vi "Servo_serial_PositionCalibration.vi"() -> ()   [LabVIEW 2017]
uses:
  <vilib>/Instr/_visa.llb/VISA Configure Serial Port (Instr).vi
panel:
  out "Servo Digital Signal":cluster{i32, dbl, dbl[]}(graph)
  out "Position Input":cluster{i32, dbl, dbl[]}(graph)
  out "Digitial Signal":dbl
  in  "Sample Rate":dbl
  in  "Buad Rate":i32(ring) items=["2400"=2400, "4800"=4800, "9600"=9600, "14400"=14400, "19200"=19200, "28800"=28800, "38400"=38400, "57600"=57600, "115200"=115200]
  out "Bytes at port":cluster{i32, dbl, dbl[]}(graph)
  out "Read buffer":string
  in  "Stop":bool
  out "Sent to Arduino":string
  in  "COM Port":refnum<visa-resource-name>
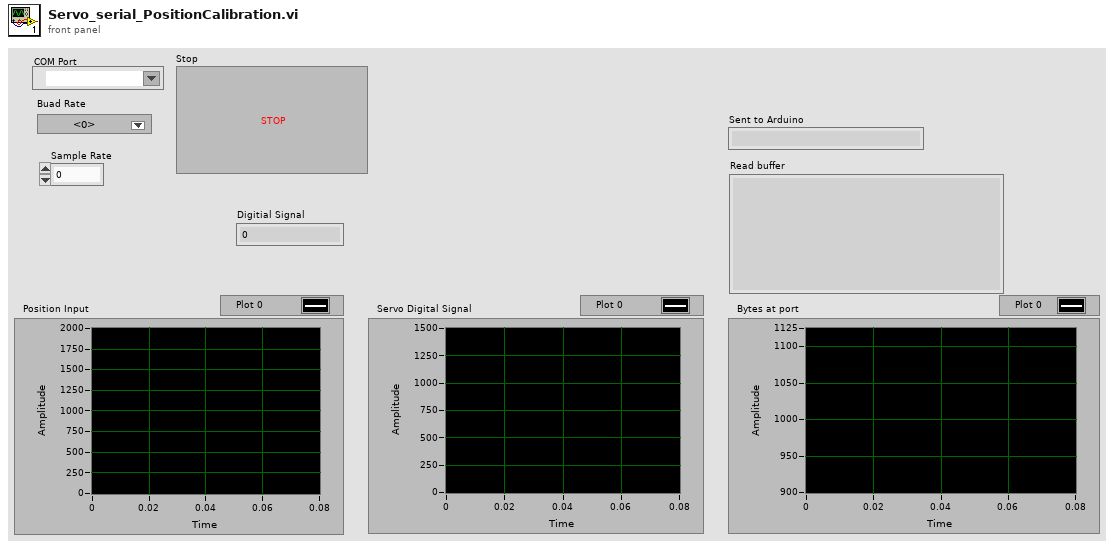
[diagram p1: front panel]
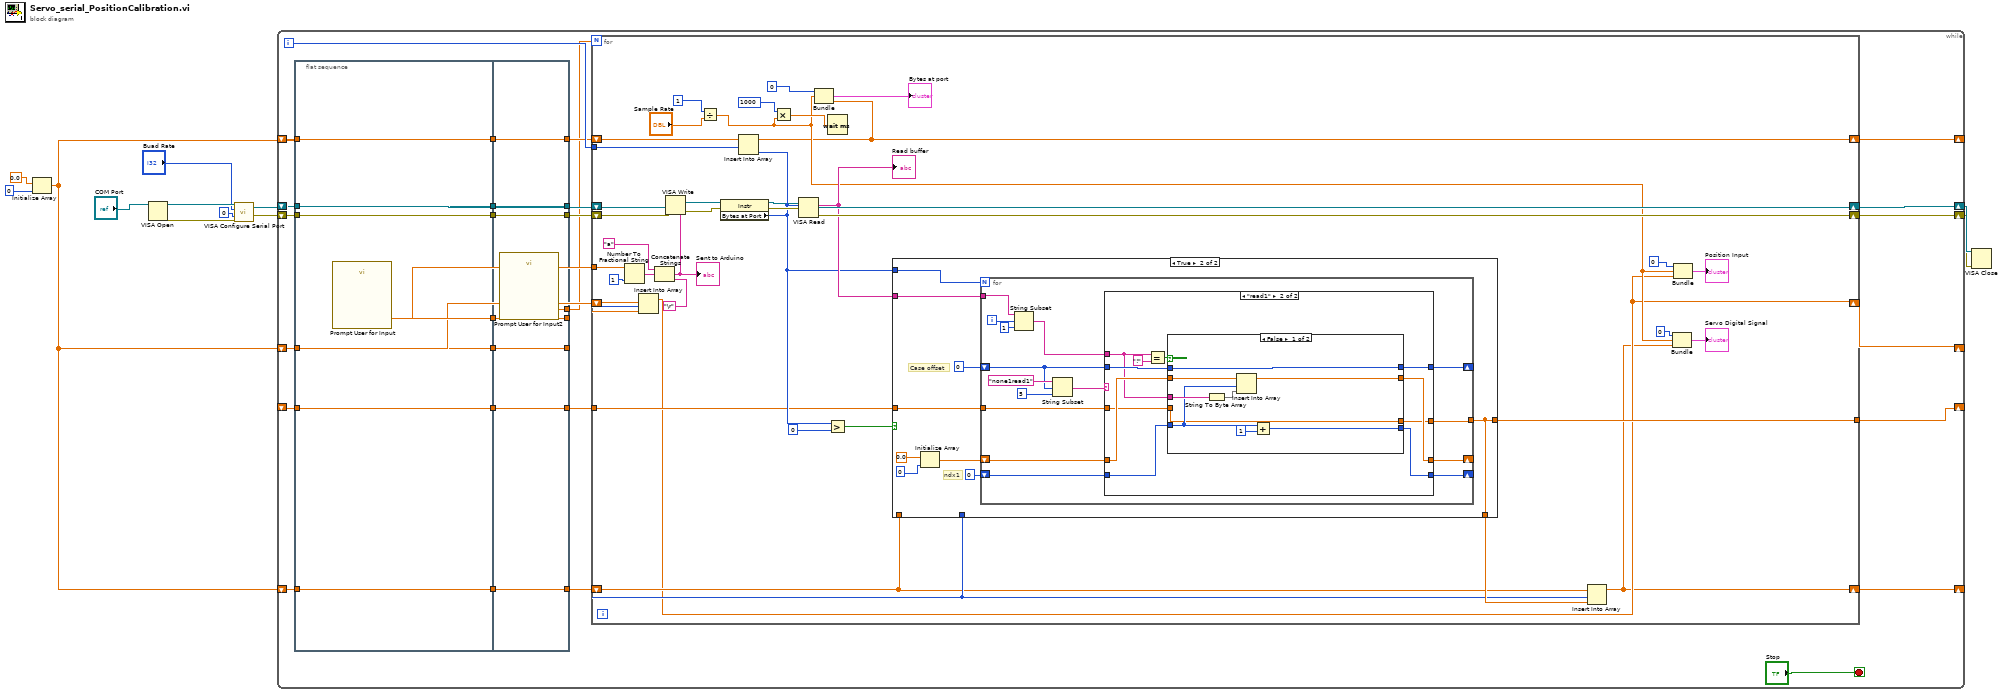
[diagram p0: block diagram]
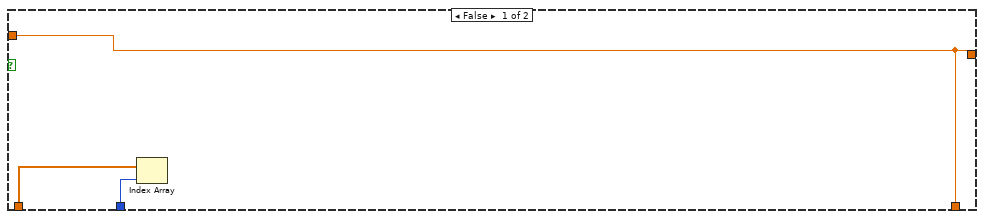
[diagram p2: hidden frame]
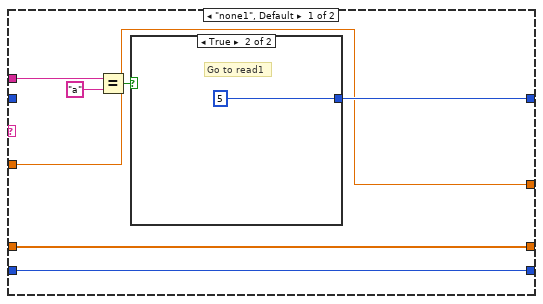
[diagram p3: hidden frame]
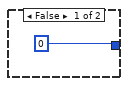
[diagram p4: hidden frame]
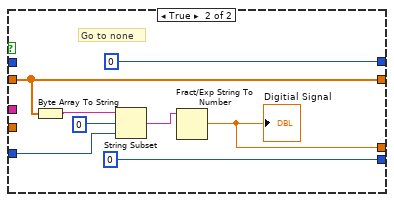
[diagram p5: hidden frame]
diagram:
  n1 = Initialize Array(0.0 ("element"), 0 ("dimension size")) -> (w7:dbl[])
  n2 = VISA Open(VISA resource name="COM Port") -> (VISA resource name=w6:refnum<visa-resource-name>, error out=w4:errorcluster)  [unwired: 4 in]
  n3 = call-poly "VISA Configure Serial Port"("VISA resource name"=w6, "baud rate (9600)"="Buad Rate", "parity (0:none)"=0, "error in (no error)"=w4) -> ("VISA resource name out"=w2:refnum<visa-resource-name>, "error out"=w3:errorcluster)  [unwired: 10 in]
  n4 = while {
    shift-right: [w36] -> w11
    shift-left: w2 -> [w30]
    shift-right: [w37] -> w10
    shift-left: w3 -> [w19]
    shift-right: [w18] -> _
    shift-left: w7 -> [w31]
    shift-right: [w17] -> _
    shift-left: w7 -> [w29]
    shift-right: [w16] -> _
    shift-left: w7 -> [w27]
    shift-right: [w32] -> _
    shift-left: _ -> [w28]
    i -> [w34]
    stop <- "Stop" stop-if-true
    n5 = flat-sequence {
      tunnel: w31 -> [w147]
      tunnel: w30 -> [w146]
      tunnel: w29 -> [w145]
      tunnel: w28 -> [w144]
      tunnel: w27 -> [w143]
      tunnel: [w142] -> w26
      tunnel: [w147] -> w25
      tunnel: [w146] -> w24
      tunnel: [w145] -> w23
      tunnel: [w144] -> w22
      tunnel: [w143] -> w21
      tunnel: [w141] -> w20
      tunnel: w19 -> [w141]
      tunnel: [w150] -> w13
      tunnel: [w151] -> w14
      tunnel: [w152] -> _
      tunnel: [w153] -> _
      tunnel: [w154] -> _
      tunnel: [w155] -> w33
      tunnel: w26 -> [w155]
      tunnel: w25 -> [w154]
      tunnel: w24 -> [w153]
      tunnel: w23 -> [w152]
      tunnel: w22 -> [w151]
      tunnel: w21 -> [w150]
      tunnel: [w149] -> _
      tunnel: w20 -> [w149]
      tunnel: [w148] -> w15
      frame #0 {
        n6 = call "Prompt User for Input"() -> ("Pulse Width"=w142:dbl)  [unwired: 17 in, 2 out]
      }
      frame #1 {
        n7 = call "Prompt User for Input2"() -> ("Number Of Trials"=w148:dbl)  [unwired: 17 in, 2 out]
      }
    }
    n8 = for {
      N: w15 -> [_]
      tunnel: w34 -> [w57]
      tunnel: w33 -> [w53]
      tunnel: [w52] -> w32
      tunnel: w14 -> [w43]
      shift-right: [w75] -> w36
      shift-left: w30 -> [w45]
      shift-right: [w76] -> w37
      shift-left: w19 -> [w41]
      shift-right: [w38] -> w16
      shift-left: w13 -> [w42]
      shift-right: [w39] -> w17
      shift-left: w29 -> [w44]
      shift-right: [w40] -> w18
      shift-left: w31 -> [w46]
      n9 = Number To Fractional String(number=w53, precision (6)=1) -> (F-format string=w73:string)  [unwired: 2 in]
      n10 = Insert Into Array(array=w44, index=w57, new element=w53) -> (w39:dbl[])
      n11 = Concatenate Strings("a", w73, "\r") -> (w74:string)
      "Sent to Arduino" <- w74
      n12 = VISA Write(VISA resource name=w45, write buffer=w74, error in (no error)=w41) -> (VISA resource name out=w68:refnum<visa-resource-name>, error out=w71:errorcluster)  [unwired: 1 out]
      n13 = Divide(x=1, y="Sample Rate") -> (x/y=w48:dbl)
      n14 = property class="Instr"(reference=w68, error in=w71) -> (reference out=w69:refnum<visa-resource-name>, error out=w70:errorcluster, "Bytes at Port"=w63:u32)
      n15 = Insert Into Array(array=w46, index=w57, new element=w63) -> (w40:dbl[])
      n16 = Multiply(x=1000, y=w48) -> (x*y=w49:dbl)
      n17 = VISA Read(VISA resource name=w69, byte count=w63, error in (no error)=w70) -> (VISA resource name out=w75:refnum<visa-resource-name>, read buffer=w65:string, error out=w76:errorcluster)  [unwired: 1 out]
      "Read buffer" <- w65
      n18 = Bundle(0, w48, w40) -> (→"Bytes at port":cluster{i32, dbl, dbl[]})  [unwired: 1 in]
      n19 = Wait (ms)(milliseconds to wait=w49) -> ()  [unwired: 1 out]
      n20 = Greater?(x=w63, y=0) -> (0:w62:bool)
      n21 = case shown="True" w62 {
        tunnel: w63 -> [_ w82]
        tunnel: w65 -> [_ w88]
        tunnel: [w77 w80] -> w58
        tunnel: w57 -> [w78 _]
        tunnel: w42 -> [w79 _]
        tunnel: w43 -> [w77 w81]
        tunnel: [w77 w80] -> w52
        frame False {
          n22 = Index Array(array=w79, index=w78) -> ()  [unwired: 1 out]
        }
        frame True {
          # "ndx1"
          # "Case offset"
          n23 = Initialize Array(0.0 ("element"), 0 ("dimension size")) -> (w83:dbl[])
          n24 = for {
            N: w82 -> [_]
            tunnel: w88 -> [w102]
            shift-right: [w98] -> _
            shift-left: 0 -> [w92]
            shift-right: [w97] -> _
            shift-left: 0 -> [w96]
            shift-right: [w94] -> _
            shift-left: w83 -> [w95]
            tunnel: w81 -> [w89]
            tunnel: [w90] -> w80
            i -> [w91]
            n25 = String Subset(string=w102, offset (0)=w91, length (rest)=1 ("length (rest)")) -> (substring=w99:string)
            n26 = String Subset(string="none1read1", offset (0)=w92, length (rest)=5 ("length (rest)")) -> (substring=w93:string)
            n27 = case shown="\"read1\"" w93 {
              tunnel: w99 -> [w110 w113]
              tunnel: [w107 w120] -> w98
              tunnel: [w106 w116] -> w97
              tunnel: w96 -> [w106 w117]
              tunnel: w95 -> [w104 w118]
              tunnel: [w104 w121] -> w94
              tunnel: w92 -> [_ w119]
              tunnel: [w105 w115] -> w90
              tunnel: w89 -> [w105 w114]
              frame "none1", Default {
                n28 = Equal?(x=w110, y="a") -> (x = y?=w108:bool)
                n29 = case shown="True" w108 {
                  tunnel: [0 5] -> w107
                  frame False {
                  }
                  frame True {
                    # "Go to read1"
                  }
                }
              }
              frame "read1" {
                n30 = Equal?(x=w113, y="!") -> (x = y?=w122:bool)
                n31 = case shown="False" w122 {
                  tunnel: [w132 0] -> w116
                  tunnel: w118 -> [w126 w136]
                  tunnel: [w130 w136] -> w121
                  tunnel: w113 -> [w129 _]
                  tunnel: [w127 0] -> w120
                  tunnel: w119 -> [w127 _]
                  tunnel: w117 -> [w125 w135]
                  tunnel: [w124 w133] -> w115
                  tunnel: w114 -> [w124 _]
                  frame False {
                    n32 = String To Byte Array(string=w129) -> (unsigned byte array=w128:u8[])
                    n33 = Insert Into Array(array=w126, index=w125, new element=w128) -> (w130:dbl[])
                    n34 = Add(x=w125, y=1) -> (x+y=w132:i32)
                  }
                  frame True {
                    # "Go to none"
                    n35 = Byte Array To String(unsigned byte array=w136) -> (string=w137:string)
                    n36 = String Subset(string=w137, offset (0)=0, length (rest)=w135) -> (substring=w134:string)
                    n37 = Fract/Exp String To Number(string=w134) -> (number=w133:dbl)  [unwired: 3 in, 1 out]
                    "Digitial Signal" <- w133
                  }
                }
              }
            }
          }
        }
      }
      n38 = Insert Into Array(array=w42, index=w57, new element=w58) -> (w38:dbl[])
      n39 = Bundle(0, w48, w38) -> (→"Servo Digital Signal":cluster{i32, dbl, dbl[]})  [unwired: 1 in]
      n40 = Bundle(0, w48, w39) -> (→"Position Input":cluster{i32, dbl, dbl[]})  [unwired: 1 in]
    }
  }
  n41 = VISA Close(VISA resource name=w11, error in (no error)=w10) -> ()  [unwired: 1 out]
